vi "CASCADE LED AND LOGO VALIDATION_PATTERN_MATCH.VI"(0 "Color Plane (Color Plane Extraction 1)":i32(ring)=1 items=["Red", "Green", "Blue", "Hue", "Saturation", "Luminance", "Value", "Intensity"], 1 "Template File Path (Pattern Locate Datum)":path=path "C:/mtp/Site_Ne_sch/Projects/DS4608_FAT/IMAGES/Datum_Right1.png", 2 "Template File Path (Pattern Match CENTER_LED)":path=path "C:/mtp/Site_Ne_sch/Projects/DS4608_FAT/IMAGES/Status LED.png", 3 "Template File Path (Pattern Matching LOGO)":path=path "C:/mtp/Site_Ne_sch/Projects/DS4608_FAT/IMAGES/Zebra_Logo.png", 7 "error in":errorcluster, 8 "Image File Path":path=path "C:/SNAPSHOT.bmp") -> (20 "Matches (Pattern Locate Datum)":T2(array[cluster]) {"Bounding Box"."y" format="%.2f"; "Bounding Box"."x" format="%.2f"; "Position"."y" format="%.2f"; "Position"."x" format="%.2f"; "Score" format="%.2f"; "Scale" format="%.2f"; "Angle" format="%.2f"}, 21 "Number of Matches (Pattern Locate Datum)":i32, 22 "Matches (Pattern Match CENTER_LED)":T2(array[cluster]) {"Bounding Box"."y" format="%.2f"; "Bounding Box"."x" format="%.2f"; "Position"."y" format="%.2f"; "Position"."x" format="%.2f"; "Score" format="%.2f"; "Scale" format="%.2f"; "Angle" format="%.2f"}, 23 "Number of Matches (Pattern Match CENTER_LED)":i32, 24 "Matches (Pattern Matching LOGO)":T2(array[cluster]) {"Bounding Box"."y" format="%.2f"; "Bounding Box"."x" format="%.2f"; "Position"."y" format="%.2f"; "Position"."x" format="%.2f"; "Score" format="%.2f"; "Scale" format="%.2f"; "Angle" format="%.2f"}, 25 "Number of Matches (Pattern Matching LOGO)":i32, 27 "error out":errorcluster)   [LabVIEW 2014]
uses:
  <vilib>/vision/NI_Vision_Development_Module.lvlib
panel:
  out "Image Out":T1(plugin-control)
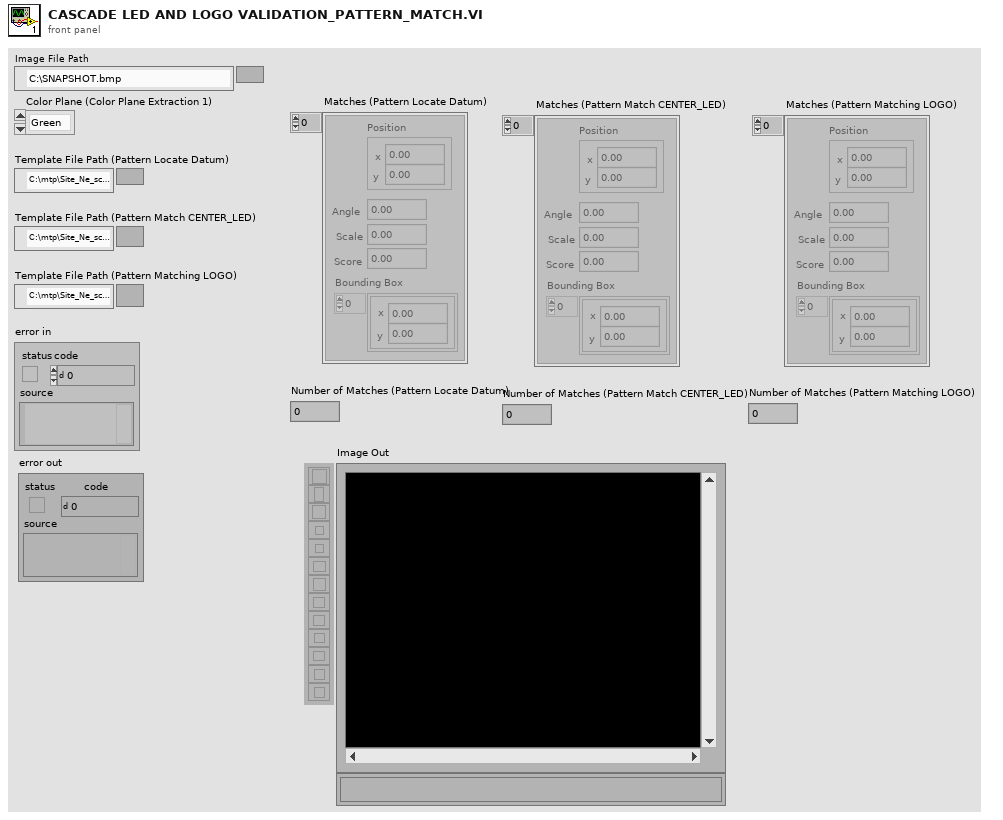
[diagram p1: front panel]
types:
  T1 = typedef "IMAQ Image.ctl" = refnum<image>
  T2 = cluster{"Position":cluster{"x":sgl, "y":sgl}, "Angle":sgl, "Scale":sgl, "Score":sgl, "Bounding Box":cluster{"x":sgl, "y":sgl}[]}[]
  T3 = cluster{"Number of Matches Requested":i32, "Minimum Match Score":sgl, "Angle Ranges":cluster{"Start Angle":sgl, "End Angle":sgl}[]}
  T4 = cluster{"Global Rectangle":i32[], "Contours":cluster{"ID":enum32{"External", "Internal"}, "Type":u32, "Coordinates":i32[]}[]}
  T5 = enum16{"Reset", "Update Coordinate System", "Get Coordinate System"}
  T6 = enum16{"Horizontal Motion", "Vertical Motion", "Horizontal and Vertical Motion", "Horizontal, Vertical and Angular Motion"}
  T7 = cluster{"Origin":cluster{"X":sgl, "Y":sgl}, "Angle (deg)":sgl, "Axis Reference":u32}
  T8 = typedef "Image Type" = u32
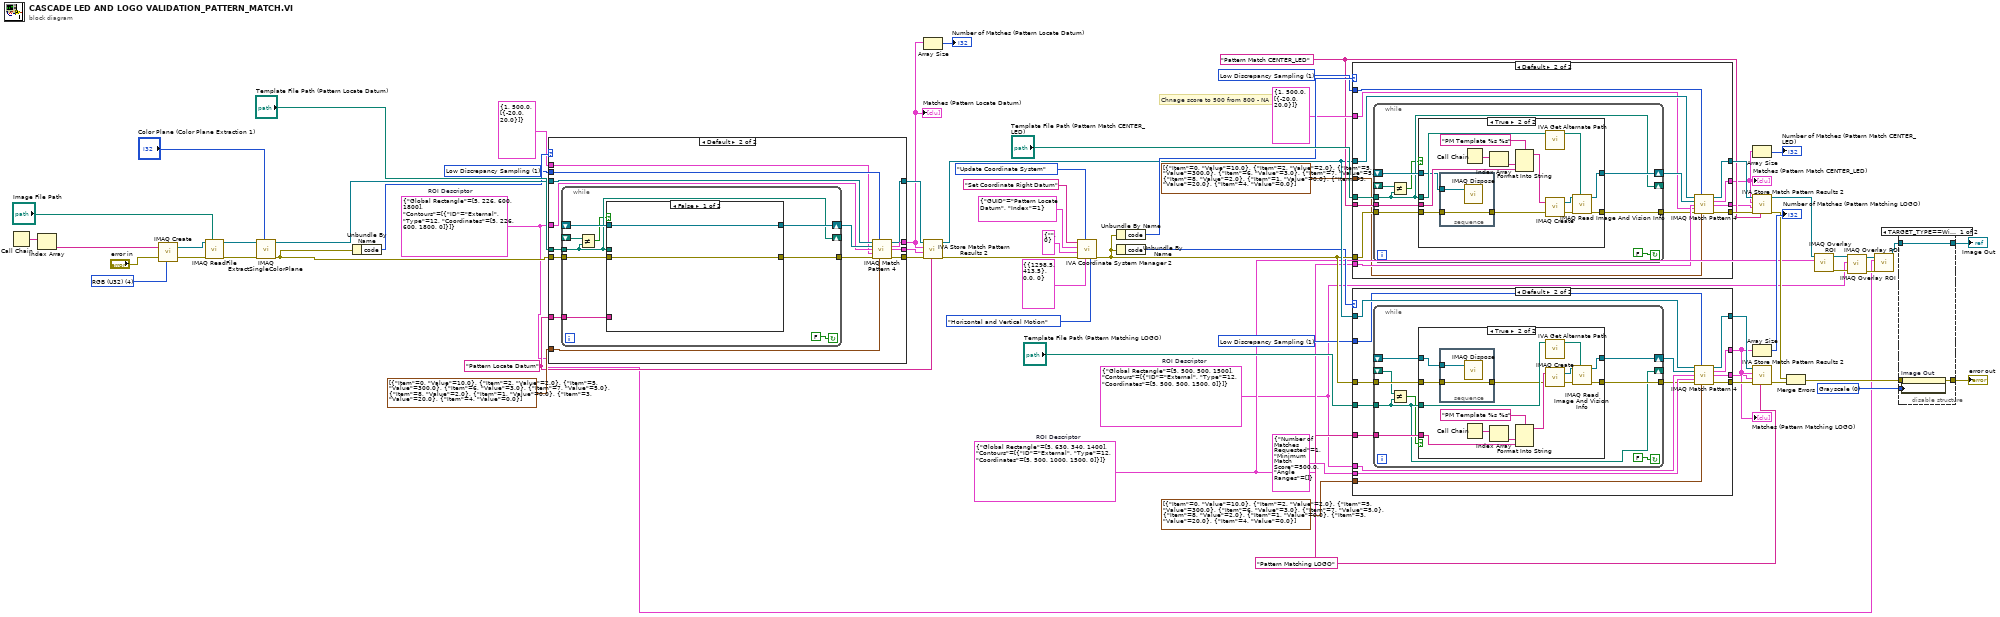
[diagram p0: block diagram]
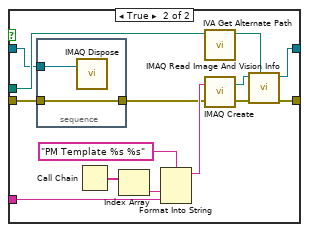
[diagram p8: hidden frame]
diagram:
  w11 = u32 0 items=["Grayscale", "Binary", "Gradient", "Rainbow", "Temperature", "User Defined"] ("Palette")
  w23 = 1 items=["All", "Low Discrepancy Sampling", "Grayscale Value Pyramid", "Gradients Pyramid"] ("Algorithm")
  w19 = "Pattern Matching LOGO" ("Step Name")
  w6 = T4 {"Global Rectangle"=[5, 500, 500, 1500], "Contours"=[{"ID"=enum."External", "Type"=12, "Coordinates"=[5, 500, 500, 1500, 0]}]}  # ROI Descriptor
  w36 = 1 items=["All", "Low Discrepancy Sampling", "Grayscale Value Pyramid", "Gradients Pyramid"] ("Algorithm")
  w32 = "Pattern Match CENTER_LED" ("Step Name")
  w9 = T4 {"Global Rectangle"=[5, 630, 340, 1400], "Contours"=[{"ID"=enum."External", "Type"=12, "Coordinates"=[5, 500, 1000, 1500, 0]}]}  # ROI Descriptor
  w54 = 1 items=["All", "Low Discrepancy Sampling", "Grayscale Value Pyramid", "Gradients Pyramid"] ("Algorithm")
  w50 = "Pattern Locate Datum" ("Step Name")
  w1 = T4 {"Global Rectangle"=[5, 226, 600, 1800], "Contours"=[{"ID"=enum."External", "Type"=12, "Coordinates"=[5, 226, 600, 1800, 0]}]}  # ROI Descriptor
  w64 = T8 4 items=["Grayscale (U8)", "Grayscale (I16)", "Grayscale (SGL)", "Complex (CSG)", "RGB (U32)", "HSL (U32)", "RGB (U64)", "Grayscale (U16)"] ("Image Type")
  # "Chnage score to 500 from 800 - NA"
  n1 = Call Chain() -> (call chain=w66:string[])
  n2 = Index Array(array=w66) -> (element=w65:string)  [unwired: 1 in]
  n3 = call "IMAQ Create"("Image Name"=w65, "Image Type"=w64, "error in (no error)"="error in") -> ("New Image"=w69:T1, "error out"=w68:errorcluster)  [unwired: 1 in, 1 out]
  n4 = call "IMAQ ReadFile"("File Path"="Image File Path", "error in (no error)"=w68, "Image"=w69) -> ("error out"=w61:errorcluster, "Image Out"=w62:T1)  [unwired: 2 in, 5 out]
  n5 = call "IMAQ ExtractSingleColorPlane"("Color Plane"="Color Plane (Color Plane Extraction 1)", "error in (no error)"=w61, "Image Src"=w62) -> ("error out"=w56:errorcluster, "Image Dst Out"=w59:T1)  [unwired: 1 in, 6 out]
  n6 = Unbundle By Name(w56) -> ("code"=w55:i32)
  n7 = case shown="Default" w55 {
    tunnel: "Template File Path (Pattern Locate Datum)" -> [_ w84]
    tunnel: w56 -> [_ w83]
    tunnel: w59 -> [w70 w78]
    tunnel: [_ w79] -> w58
    tunnel: [_ w80] -> w49
    tunnel: [w70 w77] -> w57
    tunnel: w50 -> [_ w82]
    tunnel: w54 -> [_ w76]
    tunnel: w1 -> [_ w75]
    tunnel: T3 {"Number of Matches Requested"=1, "Minimum Match Score"=500.0, "Angle Ranges"=[{"Start Angle"=-20.0, "End Angle"=20.0}]} ("Parameters") -> [_ w74]
    tunnel: cluster{"Item":u16, "Value":dbl}[] [{"Item"=0, "Value"=10.0}, {"Item"=2, "Value"=2.0}, {"Item"=5, "Value"=300.0}, {"Item"=6, "Value"=3.0}, {"Item"=7, "Value"=5.0}, {"Item"=8, "Value"=2.0}, {"Item"=1, "Value"=0.0}, {"Item"=3, "Value"=20.0}, {"Item"=4, "Value"=0.0}] ("Advanced Options") -> [_ w72]
    tunnel: [_ w71] -> w48
    frame -1074396199, -1074396198 {
      # "Discard Coordinate System Error"
    }
    frame Default {
      n8 = while {
        shift-right: [w93] -> w81
        shift-left: _ -> [w92]
        tunnel: [w90] -> w73
        tunnel: w83 -> [w89]
        tunnel: w84 -> [w86]
        tunnel: w82 -> [w88]
        shift-right: [w86] -> _
        shift-left: _ -> [w87]
        stop <- FALSE continue-if-true
        n9 = Not Equal?(x=w87, y=w86) -> (x != y?=w85:bool)
        n10 = case shown="False" w85 {
          tunnel: [w95 w107] -> w93
          tunnel: w92 -> [w95 w98]
          tunnel: [w94 w104] -> w90
          tunnel: w89 -> [w94 w97]
          tunnel: w86 -> [_ w100]
          tunnel: w88 -> [_ w101]
          frame False {
          }
          frame True {
            n11 = stacked-sequence {
              tunnel: w98 -> [w111]
              tunnel: w97 -> [w110]
              tunnel: [w110] -> w96
              frame #0 {
                n12 = call "IMAQ Dispose"("Image"=w111) -> ()  [unwired: 2 in, 4 out]
              }
            }
            n13 = Call Chain() -> (call chain=w103:string[])
            n14 = Index Array(array=w103) -> (element=w102:string)  [unwired: 1 in]
            n15 = Format Into String(format string="PM Template %s %s" ("Image Name"), w102, w101) -> (resulting string=w109:string)  [unwired: 2 in, 1 out]
            n16 = call <vilib>:"IVA Get Alternate Path.vi"("Path In"=w100) -> ("Path Out"=w99:path)  [unwired: 10 out]
            n17 = call "IMAQ Create"("Image Name"=w109, "error in (no error)"=w96) -> ("New Image"=w106:T1, "error out"=w105:errorcluster)  [unwired: 2 in, 1 out]
            n18 = call "IMAQ Read Image And Vision Info"("File Path"=w99, "error in (no error)"=w105, "Image"=w106) -> ("error out"=w104:errorcluster, "Image Out"=w107:T1)  [unwired: 1 in, 6 out]
          }
        }
      }
      n19 = call "IMAQ Match Pattern 4"("Image"=w78, "Algorithm"=w76, "Template Image"=w81, "ROI Descriptor"=w75, "Parameters"=w74, "error in (no error)"=w73, "Advanced Options"=w72) -> ("Image (duplicate)"=w77:T1, "Matches (pixel)"=w80:T2, "Matches (real-world)"=w71:T2, "error out"=w79:errorcluster)  [unwired: 4 in, 1 out]
    }
  }
  "Matches (Pattern Locate Datum)" <- w49
  n20 = Array Size(array=w49) -> (size(s)=→"Number of Matches (Pattern Locate Datum)":i32)
  n21 = call <vilib>:"IVA Store Match Pattern Results 2.vi"("Step Name"=w50, "error in (no error)"=w58, "Matches (real-world)"=w48, "Matches (pixel)"=w49, "Image in"=w57) -> ("error out"=w41:errorcluster, "Image dup"=w28:T1)  [unwired: 1 in, 4 out]
  n22 = call <vilib>:"IVA Coordinate System Manager 2.vi"("Mode"=T6."Horizontal and Vertical Motion", "Reference System"=T7 {"Origin"={"X"=1298.5, "Y"=413.5}, "Angle (deg)"=0.0, "Axis Reference"=0}, "Function"=T5."Update Coordinate System", "error in (no error)"=w41, "Angle ID"=cluster{"GUID":string, "Index":i32} {"GUID"="", "Index"=0}, "Origin ID"=cluster{"GUID":string, "Index":i32} {"GUID"="Pattern Locate Datum", "Index"=1}, "Coordinate System Name"="Set Coordinate Right Datum") -> ("error out"=w25:errorcluster)  [unwired: 4 out]
  n23 = Unbundle By Name(w25) -> ("code"=w37:i32)
  n24 = Unbundle By Name(w25) -> ("code"=w24:i32)
  n25 = case shown="Default" w37 {
    tunnel: "Template File Path (Pattern Match CENTER_LED)" -> [_ w126]
    tunnel: w25 -> [_ w125]
    tunnel: w28 -> [w112 w120]
    tunnel: [_ w121] -> w39
    tunnel: [_ w122] -> w31
    tunnel: [w112 w119] -> w38
    tunnel: w32 -> [_ w124]
    tunnel: w36 -> [_ w118]
    tunnel: w9 -> [_ w117]
    tunnel: T3 {"Number of Matches Requested"=1, "Minimum Match Score"=500.0, "Angle Ranges"=[{"Start Angle"=-20.0, "End Angle"=20.0}]} ("Parameters") -> [_ w116]
    tunnel: cluster{"Item":u16, "Value":dbl}[] [{"Item"=0, "Value"=10.0}, {"Item"=2, "Value"=2.0}, {"Item"=5, "Value"=300.0}, {"Item"=6, "Value"=3.0}, {"Item"=7, "Value"=5.0}, {"Item"=8, "Value"=2.0}, {"Item"=1, "Value"=0.0}, {"Item"=3, "Value"=20.0}, {"Item"=4, "Value"=0.0}] ("Advanced Options") -> [_ w114]
    tunnel: [_ w113] -> w30
    frame -1074396199, -1074396198 {
      # "Discard Coordinate System Error"
    }
    frame Default {
      n26 = while {
        shift-right: [w135] -> w123
        shift-left: _ -> [w134]
        tunnel: [w132] -> w115
        tunnel: w125 -> [w131]
        tunnel: w126 -> [w128]
        tunnel: w124 -> [w130]
        shift-right: [w128] -> _
        shift-left: _ -> [w129]
        stop <- FALSE continue-if-true
        n27 = Not Equal?(x=w129, y=w128) -> (x != y?=w127:bool)
        n28 = case shown="True" w127 {
          tunnel: [w137 w149] -> w135
          tunnel: w134 -> [w137 w140]
          tunnel: [w136 w146] -> w132
          tunnel: w131 -> [w136 w139]
          tunnel: w128 -> [_ w142]
          tunnel: w130 -> [_ w143]
          frame False {
          }
          frame True {
            n29 = stacked-sequence {
              tunnel: w140 -> [w153]
              tunnel: w139 -> [w152]
              tunnel: [w152] -> w138
              frame #0 {
                n30 = call "IMAQ Dispose"("Image"=w153) -> ()  [unwired: 2 in, 4 out]
              }
            }
            n31 = Call Chain() -> (call chain=w145:string[])
            n32 = Index Array(array=w145) -> (element=w144:string)  [unwired: 1 in]
            n33 = Format Into String(format string="PM Template %s %s" ("Image Name"), w144, w143) -> (resulting string=w151:string)  [unwired: 2 in, 1 out]
            n34 = call <vilib>:"IVA Get Alternate Path.vi"("Path In"=w142) -> ("Path Out"=w141:path)  [unwired: 10 out]
            n35 = call "IMAQ Create"("Image Name"=w151, "error in (no error)"=w138) -> ("New Image"=w148:T1, "error out"=w147:errorcluster)  [unwired: 2 in, 1 out]
            n36 = call "IMAQ Read Image And Vision Info"("File Path"=w141, "error in (no error)"=w147, "Image"=w148) -> ("error out"=w146:errorcluster, "Image Out"=w149:T1)  [unwired: 1 in, 6 out]
          }
        }
      }
      n37 = call "IMAQ Match Pattern 4"("Image"=w120, "Algorithm"=w118, "Template Image"=w123, "ROI Descriptor"=w117, "Parameters"=w116, "error in (no error)"=w115, "Advanced Options"=w114) -> ("Image (duplicate)"=w119:T1, "Matches (pixel)"=w122:T2, "Matches (real-world)"=w113:T2, "error out"=w121:errorcluster)  [unwired: 4 in, 1 out]
    }
  }
  "Matches (Pattern Match CENTER_LED)" <- w31
  n38 = case shown="Default" w24 {
    tunnel: "Template File Path (Pattern Matching LOGO)" -> [_ w168]
    tunnel: w25 -> [_ w167]
    tunnel: w28 -> [w154 w162]
    tunnel: [_ w163] -> w27
    tunnel: [_ w164] -> w18
    tunnel: [w154 w161] -> w26
    tunnel: w19 -> [_ w166]
    tunnel: w23 -> [_ w160]
    tunnel: w6 -> [_ w159]
    tunnel: T3 {"Number of Matches Requested"=1, "Minimum Match Score"=500.0, "Angle Ranges"=[]} ("Parameters") -> [_ w158]
    tunnel: cluster{"Item":u16, "Value":dbl}[] [{"Item"=0, "Value"=10.0}, {"Item"=2, "Value"=2.0}, {"Item"=5, "Value"=300.0}, {"Item"=6, "Value"=3.0}, {"Item"=7, "Value"=5.0}, {"Item"=8, "Value"=2.0}, {"Item"=1, "Value"=0.0}, {"Item"=3, "Value"=20.0}, {"Item"=4, "Value"=0.0}] ("Advanced Options") -> [_ w156]
    tunnel: [_ w155] -> w17
    frame -1074396199, -1074396198 {
      # "Discard Coordinate System Error"
    }
    frame Default {
      n39 = while {
        shift-right: [w177] -> w165
        shift-left: _ -> [w176]
        tunnel: [w174] -> w157
        tunnel: w167 -> [w173]
        tunnel: w168 -> [w170]
        tunnel: w166 -> [w172]
        shift-right: [w170] -> _
        shift-left: _ -> [w171]
        stop <- FALSE continue-if-true
        n40 = Not Equal?(x=w171, y=w170) -> (x != y?=w169:bool)
        n41 = case shown="True" w169 {
          tunnel: [w179 w191] -> w177
          tunnel: w176 -> [w179 w182]
          tunnel: [w178 w188] -> w174
          tunnel: w173 -> [w178 w181]
          tunnel: w170 -> [_ w184]
          tunnel: w172 -> [_ w185]
          frame False {
          }
          frame True {
            n42 = stacked-sequence {
              tunnel: w182 -> [w195]
              tunnel: w181 -> [w194]
              tunnel: [w194] -> w180
              frame #0 {
                n43 = call "IMAQ Dispose"("Image"=w195) -> ()  [unwired: 2 in, 4 out]
              }
            }
            n44 = Call Chain() -> (call chain=w187:string[])
            n45 = Index Array(array=w187) -> (element=w186:string)  [unwired: 1 in]
            n46 = Format Into String(format string="PM Template %s %s" ("Image Name"), w186, w185) -> (resulting string=w193:string)  [unwired: 2 in, 1 out]
            n47 = call <vilib>:"IVA Get Alternate Path.vi"("Path In"=w184) -> ("Path Out"=w183:path)  [unwired: 10 out]
            n48 = call "IMAQ Create"("Image Name"=w193, "error in (no error)"=w180) -> ("New Image"=w190:T1, "error out"=w189:errorcluster)  [unwired: 2 in, 1 out]
            n49 = call "IMAQ Read Image And Vision Info"("File Path"=w183, "error in (no error)"=w189, "Image"=w190) -> ("error out"=w188:errorcluster, "Image Out"=w191:T1)  [unwired: 1 in, 6 out]
          }
        }
      }
      n50 = call "IMAQ Match Pattern 4"("Image"=w162, "Algorithm"=w160, "Template Image"=w165, "ROI Descriptor"=w159, "Parameters"=w158, "error in (no error)"=w157, "Advanced Options"=w156) -> ("Image (duplicate)"=w161:T1, "Matches (pixel)"=w164:T2, "Matches (real-world)"=w155:T2, "error out"=w163:errorcluster)  [unwired: 4 in, 1 out]
    }
  }
  "Matches (Pattern Matching LOGO)" <- w18
  n51 = Array Size(array=w31) -> (size(s)=→"Number of Matches (Pattern Match CENTER_LED)":i32)
  n52 = call <vilib>:"IVA Store Match Pattern Results 2.vi"("Step Name"=w32, "error in (no error)"=w39, "Matches (real-world)"=w30, "Matches (pixel)"=w31, "Image in"=w38) -> ("error out"=w16:errorcluster, "Image dup"=w5:T1)  [unwired: 1 in, 4 out]
  n53 = Array Size(array=w18) -> (size(s)=→"Number of Matches (Pattern Matching LOGO)":i32)
  n54 = call <vilib>:"IVA Store Match Pattern Results 2.vi"("Step Name"=w19, "error in (no error)"=w27, "Matches (real-world)"=w17, "Matches (pixel)"=w18, "Image in"=w26) -> ("error out"=w15:errorcluster)  [unwired: 1 in, 5 out]
  n55 = Merge Errors(w16, w15) -> (w14:errorcluster)
  n56 = call "IMAQ Overlay ROI"("ROI Descriptor"=w9, "Image"=w5) -> ("error out"=w8:errorcluster, "Image Out"=w7:T1)  [unwired: 8 in]
  n57 = call "IMAQ Overlay ROI"("error in (no error)"=w8, "ROI Descriptor"=w6, "Image"=w7) -> ("error out"=w4:errorcluster, "Image Out"=w3:T1)  [unwired: 7 in]
  n58 = call "IMAQ Overlay ROI"("error in (no error)"=w4, "ROI Descriptor"=w1, "Image"=w3) -> ("Image Out"=w2:T1)  [unwired: 7 in, 1 out]
  n59 = disable-structure "Conditional Disable Structure" shown="TARGET_TYPE==Windows" {
    disable-tunnel: w14 -> [w199 w200]
    disable-tunnel: [w198 w200] -> w13
    disable-tunnel: w2 -> [w197 w201]
    disable-tunnel: [w197 w201] -> w12
    disable-tunnel: w11 -> [w196 _]
    frame condition #0 (active) {
      n60 = property on="Image Out" class="ImageControl"(error in=w199, "Palette:Palette Type"=w196) -> (error out=w198:errorcluster)  [unwired: 1 in, 1 out]
    }
    frame condition #1 {
    }
  }
  "error out" <- w13
  "Image Out" <- w12
